vi "obj_LuaVIEW Task Preparations.vi"(0 "method":T5=enum."empty", 7 "script infos in":T1[](array[typedef]), 11 "task info in":T2 {"handle mask" format="%.0b"; "allow mask" format="%.0b"; "signal flags" format="%.0b"}) -> (4 "empty?":bool, 8 "script infos out":T1[](array[typedef]), 15 "task info out":T2 {"handle mask" format="%.0b"; "allow mask" format="%.0b"; "signal flags" format="%.0b"})   [LabVIEW 2012]
doc: "Serves to pass initialisation data to a newly started task. Preparations for further tasks do not commence until this object is emptied, or its contents discarded. This, in conjunction with the \"Task State Instantiator\" object, ensures that the actions of \"Do Task\", \"Run Task\", and \"Swap Task\" are properly mutexed.\n\nIt would have been more elegant to instantiate and adorn a task state object and hand that over to the task. However, to guarantee [1] that the object remains open as long as the task lives, it would have to be instantiated in the top-level context of the task thus leading to a chicken-and-egg problem.\n\n[1] LabVIEW's ill-conceived resource tracking closes VI references when the top level context that opened them completes\n\nPreviously, this issue was circumvented via an object template inside the task. This triggers co-instantiation on task instantiation (before it was run). This technique was dropped because templates are far more expensive to instantiate than a pre-loaded reentrant VI."
uses:
  typedefs/clusters/LuaVIEW Script Info.ctl
  typedefs/t_LuaVIEW Prepared Script Infos Methods.ctl
  typedefs/clusters/LuaVIEW Task Info.ctl
  typedefs/t_LuaVIEW Task Modes.ctl
  typedefs/t_LuaVIEW Reference.ctl
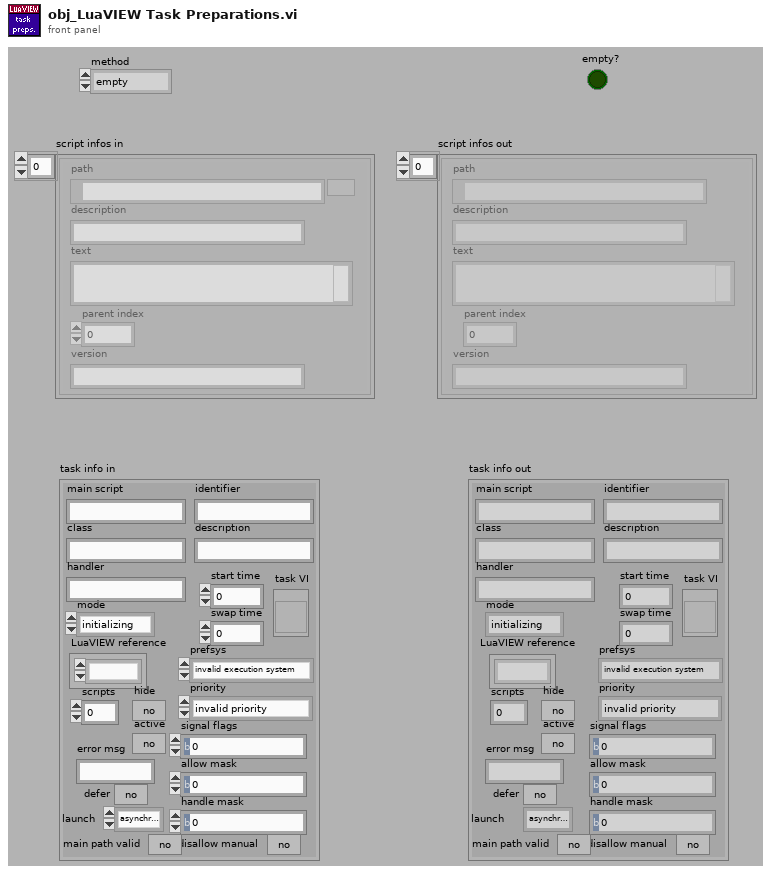
[diagram p1: front panel]
types:
  T1 = typedef "LuaVIEW Script Info.ctl" = cluster{"path":path, "description":string, "text":string, "parent index":i32, "version":string}
  T2 = typedef "LuaVIEW Task Info.ctl" = cluster{"main script":string, "identifier":string, "class":string, "description":string, "mode":T3, "handler":string, "LuaVIEW reference":T4, "scripts":i32, "hide":bool, "active":bool, "error msg":string, "defer":bool, "launch":enum16{"asynchronous", "manual", "synchronous"}, "main path valid":bool, "start time":dbl, "swap time":dbl, "task VI":refnum<vi>, "prefsys":enum32{"invalid execution system", "user interface", "standard", "instrument i/o", "data acquisition", "other 1", "other 2", "same as caller"}, "priority":enum32{"invalid priority", "background priority", "normal priority", "above normal priority", "high priority", "time critical priority", "subroutine"}, "signal flags":u32, "allow mask":u32, "handle mask":u32, "disallow manual":bool}
  T3 = typedef "t_LuaVIEW Task Modes.ctl" = enum16{"initializing", "running", "executing", "paused", "error", "swapping"}
  T4 = typedef "t_LuaVIEW Reference.ctl" = refnum<k1>
  T5 = typedef "t_LuaVIEW Prepared Script Infos Methods.ctl" = enum16{"isempty?", "empty", "set", "discard"}
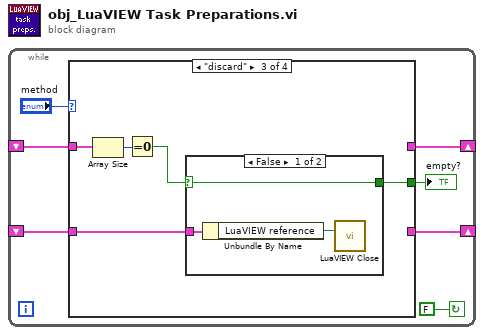
[diagram p0: block diagram]
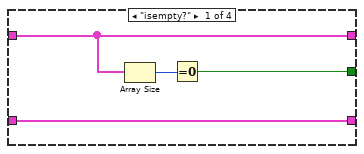
[diagram p2: hidden frame]
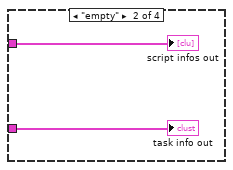
[diagram p3: hidden frame]
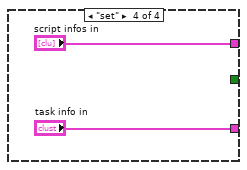
[diagram p5: hidden frame]
diagram:
  n1 = while {
    shift-right: [w4] -> _
    shift-left: _ -> [w5]
    shift-right: [w3] -> _
    shift-left: _ -> [w2]
    stop <- FALSE continue-if-true
    n2 = case shown="\"discard\"" "method" {
      tunnel: w5 -> [w9 w13 w16 _]
      tunnel: [w9 _ _ "script infos in"] -> w4
      tunnel: [w11 _ _ "task info in"] -> w3
      tunnel: w2 -> [w11 w12 w18 _]
      tunnel: [w8 _ w15 _] -> w1
      frame "isempty?" {
        n3 = Array Size(array=w9) -> (size(s)=w10:i32)
        n4 = Equal To 0?(x=w10) -> (x = 0?=w8:bool)
      }
      frame "empty" {
        "task info out" <- w12
        "script infos out" <- w13
      }
      frame "discard" {
        n5 = Array Size(array=w16) -> (size(s)=w17:i32)
        n6 = Equal To 0?(x=w17) -> (x = 0?=w14:bool)
        n7 = case shown="False" w14 {
          selector: w14 -> [w19 w22]
          tunnel: w18 -> [w21 _]
          tunnel: [w19 w22] -> w15
          frame False {
            n8 = Unbundle By Name(w21) -> ("LuaVIEW reference"=w20:T4)
            n9 = call "LuaVIEW Close.vi"("LuaVIEW reference"=w20) -> ()  [unwired: 14 in, 1 out]
          }
          frame True {
          }
        }
      }
      frame "set" {
      }
    }
    "empty?" <- w1
  }
